vi "Query Analog Channels.vi"(8 "error in":errorcluster, 11 "4300 in":refnum<class "4300.lvclass">) -> (0 "error out":errorcluster, 2 "Timed Out":bool, 3 "4300 out":refnum<class "4300.lvclass">)   [LabVIEW 2019, in "4300.lvlib" / "4300.lvclass"]
uses:
  Library/4300.lvclass
  C:/Users/Public/Documents/Development/builds/Instruments/AnalogInput.lvlibp/Library/AnalogInput.lvclass
  C:/Users/Public/Documents/Development/builds/Instruments/Instruments.lvlibp/Library/Instruments.lvclass
  Library/4300.lvclass/4300.ctl
  <vilib>/DAQmx/read.llb/DAQmx Read (Analog 1D Wfm NChan NSamp).vi
  builds/Instruments/AnalogInput.lvlibp/Accessors/Triggering/Read Trigger Settings.vi
  <vilib>/DAQmx/miscellaneous.llb/DAQmx Fill In Error Info.vi
  builds/Instruments/Instruments.lvlibp/Accessors/Write Measured.vi
  builds/Instruments/AnalogInput.lvlibp/Accessors/Write Timeout Event.vi
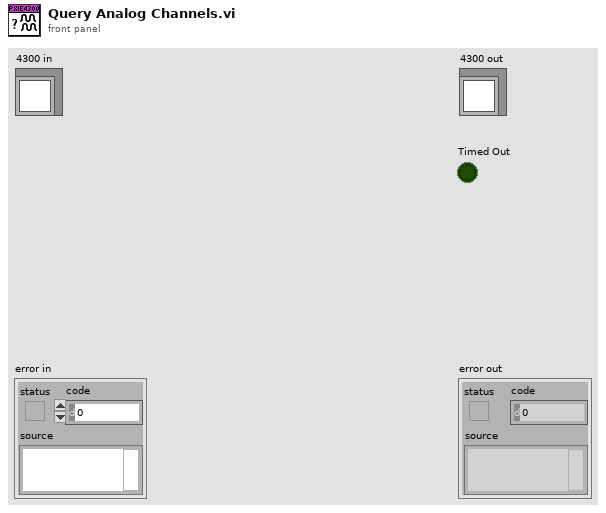
[diagram p1: front panel]
types:
  T1 = typedef "AnalogInput.lvlibp/AnalogInput.lvclass/User Trigger Settings.ctl" = cluster{"Timeout":dbl, "Level":dbl, "Slope":T2, "samples per channel":i32, "Sample Rate (10k)":dbl, "pretrigger samples":u32}
  T2 = typedef "AnalogInput.lvlibp/AnalogInput.lvclass/Trigger_Slope.ctl" = enum16{"Rising", "Falling"}
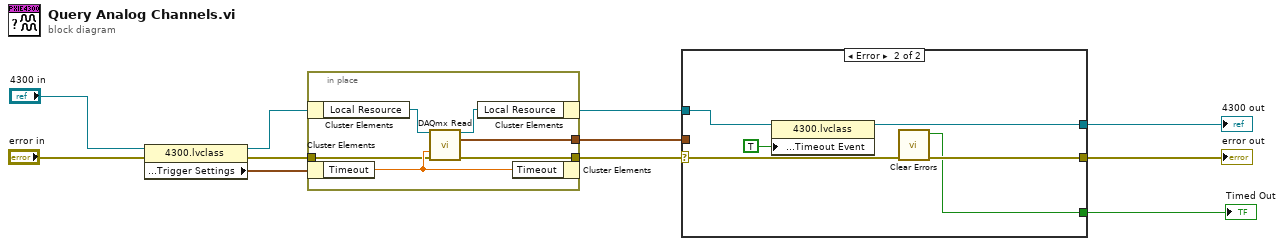
[diagram p0: block diagram]
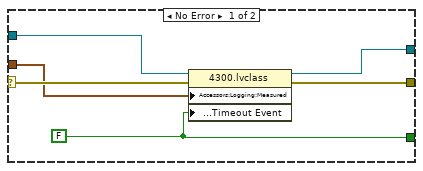
[diagram p2: hidden frame]
diagram:
  n1 = property class="4300.lvclass"(reference="4300 in", error in="error in") -> (reference out=w3:refnum<class "4300.lvclass">, error out=w2:errorcluster, "Accessors:Triggering:Trigger Settings"=w6:T1)
  n2 = in-place {
    in-place-border: [w14] -> w4
    in-place-border: [w13] -> w1
    in-place-border: w2 -> [w12]
    n3 = in-place-cluster #1(w3) -> ("Local Resource"=w17:refnum<k21>)
    n4 = in-place-cluster #2(w6) -> ("Timeout"=w15:dbl)
    n5 = call-poly <vilib>:"DAQmx Read.vi"("task/channels in"=w17, "timeout"=w15, "error in"=w12) -> ("task out"=w16:refnum<k21>, "data"=w14:waveform(dbl)[], "error out"=w13:errorcluster)  [unwired: 10 in]
    n6 = in-place-cluster #1("Local Resource"=w16) -> (w5:refnum<class "4300.lvclass">)
    n7 = in-place-cluster #2("Timeout"=w15) -> ()  [unwired: 1 out]
  }
  n8 = case shown="Error" w1 {
    selector: w1 -> [w22 w29]
    tunnel: w5 -> [w23 w26]
    tunnel: w4 -> [w19 _]
    tunnel: [w20 w25] -> w10
    tunnel: [w21 w28] -> w9
    tunnel: [w18 w27] -> w8
    frame No Error {
      w18 = FALSE ("Timeout Event")
      n9 = property class="4300.lvclass"(reference=w23, error in=w22, "Accessors:Logging:Measured"=w19, "Accessors:Triggering:Timeout Event"=w18) -> (reference out=w20:refnum<class "4300.lvclass">, error out=w21:errorcluster)
    }
    frame Error {
      n10 = property class="4300.lvclass"(reference=w26, "Accessors:Triggering:Timeout Event"=TRUE ("Timeout Event")) -> (reference out=w25:refnum<class "4300.lvclass">)  [unwired: 1 in, 1 out]
      n11 = call <vilib>:"Clear Errors.vi"("error in (no error)"=w29) -> ("error out"=w28:errorcluster, "specific error cleared?"=w27:bool)  [unwired: 5 in]
    }
  }
  "error out" <- w9
  "4300 out" <- w10
  "Timed Out" <- w8
